vi "txmessages raw.vi"(8 "error in (no error)":errorcluster, 9 "networkID":u8, 10 "Messages Raw In":u8[](array[numeric]) format="%.0x", 11 "hObject":i32) -> (0 "error out":errorcluster, 3 "hObject Out":i32)   [LabVIEW 2009]
doc: "this vi transmit a CAN message to the device. for Non-CAN network, use the \"TxMessages J1850.vi\".\n\n12/21/2010 1.0.0 jyg\n- initial release"
uses:
  NEO VI Example/data/icsneo40.dll
panel:
  in  "iNumMessages":i32=1
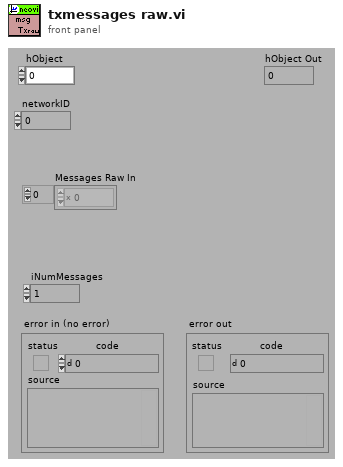
[diagram p1: front panel]
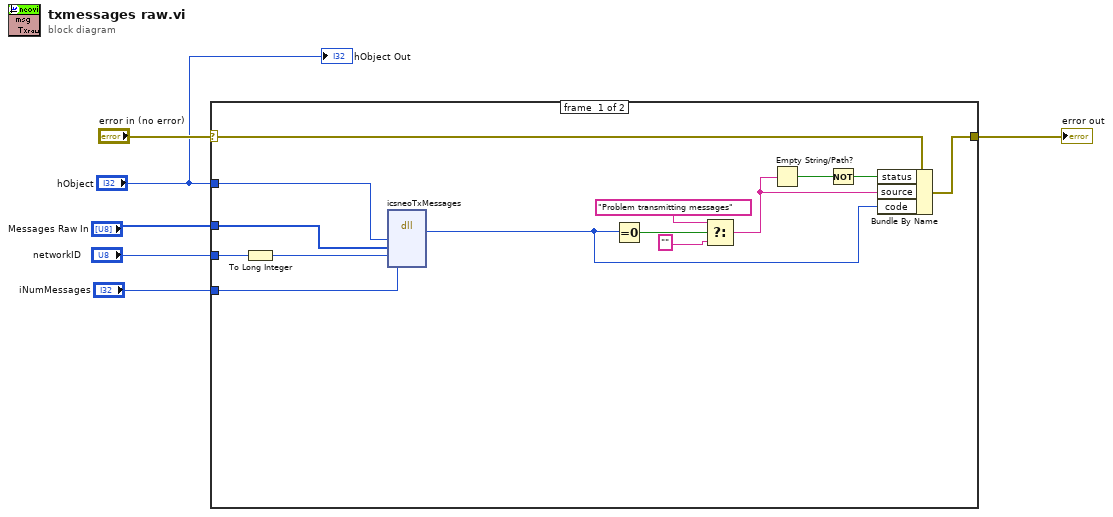
[diagram p0: block diagram]
diagram:
  n1 = case shown="No Error" "error in (no error)" {
    selector: "error in (no error)" -> [w16 w21]
    tunnel: "hObject" -> [w11 _]
    tunnel: [w17 w21] -> w6
    tunnel: "networkID" -> [w10 _]
    tunnel: "iNumMessages" -> [w8 _]
    tunnel: "Messages Raw In" -> [w7 _]
    frame #0 {
      n2 = To Long Integer(number=w10) -> (32bit integer=w9:i32)
      n3 = dll-call lib="C:/WINDOWS/system32/icsneo40.dll" fn="icsneoTxMessages"("hObject"=w11, "pMsg"=w7, "1NetworkID"=w9, "1NumMessages"=w8) -> ("return type"=w15:i32)  [unwired: 7 in, 2 out]
      n4 = Equal To 0?(x=w15) -> (x = 0?=w14:bool)
      n5 = Select(t="Problem transmitting messages", s=w14, f="") -> (s? t:f=w13:string)
      n6 = Empty String/Path?(string/path=w13) -> (empty?=w19:bool)
      n7 = Not(x=w19) -> (.not. x?=w18:bool)
      n8 = Bundle By Name(cluster=w16, "status"=w18, "source"=w13, "code"=w15) -> (w17:errorcluster)
    }
    frame #1 {
    }
  }
  "error out" <- w6
  "hObject Out" <- "hObject"
